vi "CreateUint32.vi"(6 "Numeric in":u8, 9 "Numeric 3":u8, 10 "Numeric 4":u8, 11 "Numeric 5":u8) -> (3 "Numeric out":u32)   [LabVIEW 2016]
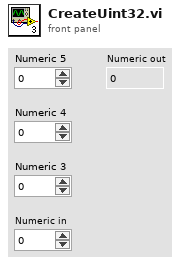
[diagram p1: front panel]
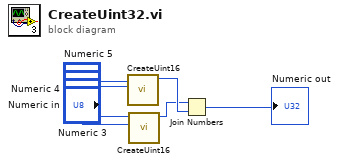
[diagram p0: block diagram]
diagram:
  n1 = call "CreateUint16.vi"("high"="Numeric 4", "low"="Numeric 5") -> ("Numeric 3"=w2:u16)  [unwired: 9 in]
  n2 = call "CreateUint16.vi"("high"="Numeric in", "low"="Numeric 3") -> ("Numeric 3"=w1:u16)  [unwired: 9 in]
  n3 = Join Numbers(hi=w1, lo=w2) -> ((hi.lo)=→"Numeric out":u32)
